vi "test_OneSessOnePinOneInstrOneSiteRes_CallGetConnFromPinsForAllDcPowerPinsAllSitesWithNoReservePins_ReturnsOneConn.vi"(8 "error in":errorcluster) -> (0 "error out":errorcluster, 2 "result":string, 3 "pass":bool)   [LabVIEW 2020, in "MeasurementServerTests.lvlib"]
uses:
  MeasurementServerTests.lvlib
  Runtime/Measurements/Measurement Plugin Session Management V1/Session Reservation/Connection with Session.ctl
  Runtime/Measurements/Measurement Plugin Session Management V1/Session Reservation/Connection.ctl
  Runtime/MeasurementLink niDCPower/Session Factory/Session Factory.lvclass
  D:/TAF/measurement-plugin-labview/Source/Runtime/MeasurementLink Instrument/ISession Factory/ISession Factory.lvclass
  Runtime/Measurements/Measurement Plugin Session Management V1/Session Reservation/Pin Type.ctl
  bc16729a-64c0-4dda-ad96-b8d210a09fe2.vi
  577716b6-6942-4938-a0b7-4602e2b65465.vi
  23f6d8a8-1a50-4614-87d2-c80af14f8c4e.vi
  <vilib>/AdvancedString/1D String Array to Delimited String.vi
  23f6d8a8-1a50-4614-87d2-c80af14f8c4e.vi/94283ac5-2298-4b3a-b57d-7be67da3787d.vi
  23f6d8a8-1a50-4614-87d2-c80af14f8c4e.vi/f7d9c9cb-0251-4d67-81cb-70e1b0e8b69f.vi
  23f6d8a8-1a50-4614-87d2-c80af14f8c4e.vi/48d9c053-c3ce-4ae4-8653-846fcb37df32.vi
  23f6d8a8-1a50-4614-87d2-c80af14f8c4e.vi/38a8d12d-9165-42a0-bd04-ad62bed472d1.vi
  Runtime/Measurements/Measurement Plugin Session Management V1/Session Reservation/Get Connections Impl.vi
  <vilib>/JDP Science/JSONtext/Variant to JSON Text.vi
  <vilib>/JDP Science/JSONtext/LVClass Serializer/JSONtext LVClass Serializer.lvclass
  Runtime/Measurements/Measurement Plugin Session Management V1/Session Reservation/Session Reservation.lvclass
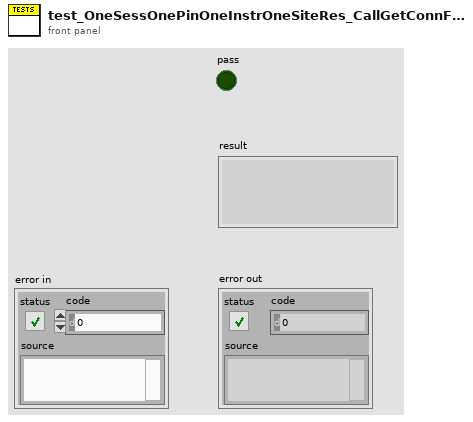
[diagram p1: front panel]
types:
  T1 = typedef "Measurement Plugin Session Management V1.lvlib/Session Reservation.lvclass/Pin Type.ctl" = enum16{"DUT and System Pins", "System Pins"}
  T2 = typedef "Measurement Plugin Session Management V1.lvlib/Session Reservation.lvclass/Connection.ctl" = cluster{"pin or relay name":string, "site":i32, "instrument type id":string, "channel":string}
  T3 = typedef "Measurement Plugin Session Management V1.lvlib/Session Reservation.lvclass/Connection with Session.ctl" = cluster{"connection":T2, "session":variant}
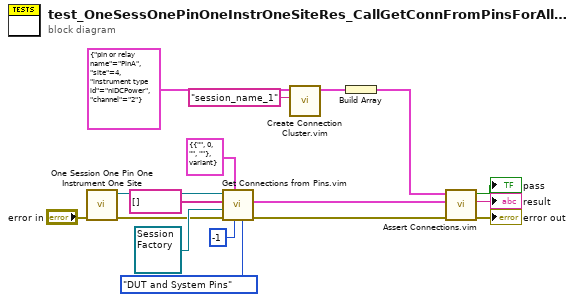
[diagram p0: block diagram]
diagram:
  n1 = call "One Session One Pin One Instrument One Site.vi"("error in"="error in") -> ("error out"=w3:errorcluster, "session reservation out"=w4:refnum<class "Session Reservation.lvclass">)  [unwired: 8 in, 1 out]
  n2 = call "Get Connections from Pins.vim"("pin type"=Pin_Type."DUT and System Pins", "site"=-1, "connection type"=T3 {"connection"={"pin or relay name"="", "site"=0, "instrument type id"="", "channel"=""}, "session"=variant} ("connection"), "error in"=w3, "session factory"=refnum<class "Session Factory.lvclass"> refnum ("MeasurementLink niDCPower.lvlib:Instrument.lvclass"), "pin or relay names"=string[] [], "session reservation in"=w4) -> ("error out"=w2:errorcluster, "connections"=w17:T3[])  [unwired: 2 in, 1 out]
  n3 = call "Create Connection Cluster.vim"("session in"="session_name_1", "hardware independent connection in"=T2 {"pin or relay name"="PinA", "site"=4, "instrument type id"="niDCPower", "channel"="2"} ("connection")) -> ("connection out"=w14:T3)  [unwired: 9 in]
  n4 = Build Array(w14) -> (w7:T3[])
  n5 = call "Assert Connections.vim"("error in"=w2, "actual connections"=w17, "expected connections"=w7) -> ("error out"=→"error out":errorcluster, "result"=→"result":string, "pass"=→"pass":bool)  [unwired: 6 in]
